vi "fxp32_to_i32-8.vi"(0 "fxp32_16":fxp<+/-,32,16>, 1 "fxp32_16 2":fxp<+/-,32,16>, 2 "fxp32_16 3":fxp<+/-,32,16>, 3 "fxp32_16 4":fxp<+/-,32,16>, 4 "fxp32_16 5":fxp<+/-,32,16>, 5 "fxp32_16 6":fxp<+/-,32,16>, 6 "fxp32_16 7":fxp<+/-,32,16>, 7 "fxp32_16 8":fxp<+/-,32,16>) -> (20 "32bit integer":i32, 21 "32bit integer 2":i32, 22 "32bit integer 3":i32, 23 "32bit integer 4":i32, 24 "32bit integer 5":i32, 25 "32bit integer 6":i32, 26 "32bit integer 7":i32, 27 "32bit integer 8":i32)   [LabVIEW 2018]
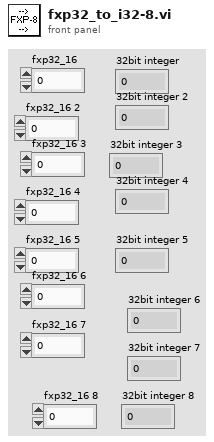
[diagram p1: front panel]
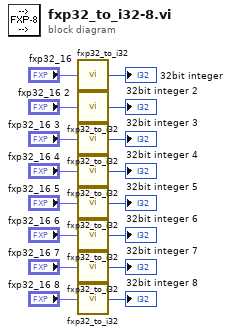
[diagram p0: block diagram]
diagram:
  n1 = call "fxp32_to_i32.vi"("fxp32_16"="fxp32_16") -> ("32bit integer"=→"32bit integer":i32)
  n2 = call "fxp32_to_i32.vi"("fxp32_16"="fxp32_16 2") -> ("32bit integer"=→"32bit integer 2":i32)
  n3 = call "fxp32_to_i32.vi"("fxp32_16"="fxp32_16 3") -> ("32bit integer"=→"32bit integer 3":i32)
  n4 = call "fxp32_to_i32.vi"("fxp32_16"="fxp32_16 4") -> ("32bit integer"=→"32bit integer 4":i32)
  n5 = call "fxp32_to_i32.vi"("fxp32_16"="fxp32_16 5") -> ("32bit integer"=→"32bit integer 5":i32)
  n6 = call "fxp32_to_i32.vi"("fxp32_16"="fxp32_16 6") -> ("32bit integer"=→"32bit integer 6":i32)
  n7 = call "fxp32_to_i32.vi"("fxp32_16"="fxp32_16 7") -> ("32bit integer"=→"32bit integer 7":i32)
  n8 = call "fxp32_to_i32.vi"("fxp32_16"="fxp32_16 8") -> ("32bit integer"=→"32bit integer 8":i32)
